vi "全局变量.vi"() -> ()   [LabVIEW 2022 SP3, in "重金属.lvlib"]
panel:
  out "连接配置":T1={"连接类型"=enum."串口", "串口"="", "IP"="192.168.1.205", "PORT"="502"}
  in  "监测值":dbl[](array[numeric])
  in  "因子编码":string[](array[string])=["w20120", "w20115", "w20122", "w20123", "w20121", "w20124", "w20111"]
  in  "参数选择配置":T2 {"通道4" items=["不启用", "铅", "镉", "铜", "锌", "镍", "锰", "汞"]; "通道3" items=["不启用", "铅", "镉", "铜", "锌", "镍", "锰", "汞"]; "通道2" items=["不启用", "铅", "镉", "铜", "锌", "镍", "锰", "汞"]; "通道1" items=["不启用", "铅", "镉", "铜", "锌", "镍", "锰", "汞"]}
  in  "参数名称table":string[](array[string])=["铅", "镉", "铜", "锌"]
  in  "测试时间设置":dbl=3600.0
  in  "运行模式":enum16{"维护模式", "常规模式", "应急模式", "质控模式", "性能测试"}(ring)
  # "w20120\t铅"
  # "w20115\t镉"
  # "w20122\t铜\nw20123\t锌"
  # "铅   镉  铜  锌  镍  锰  汞"
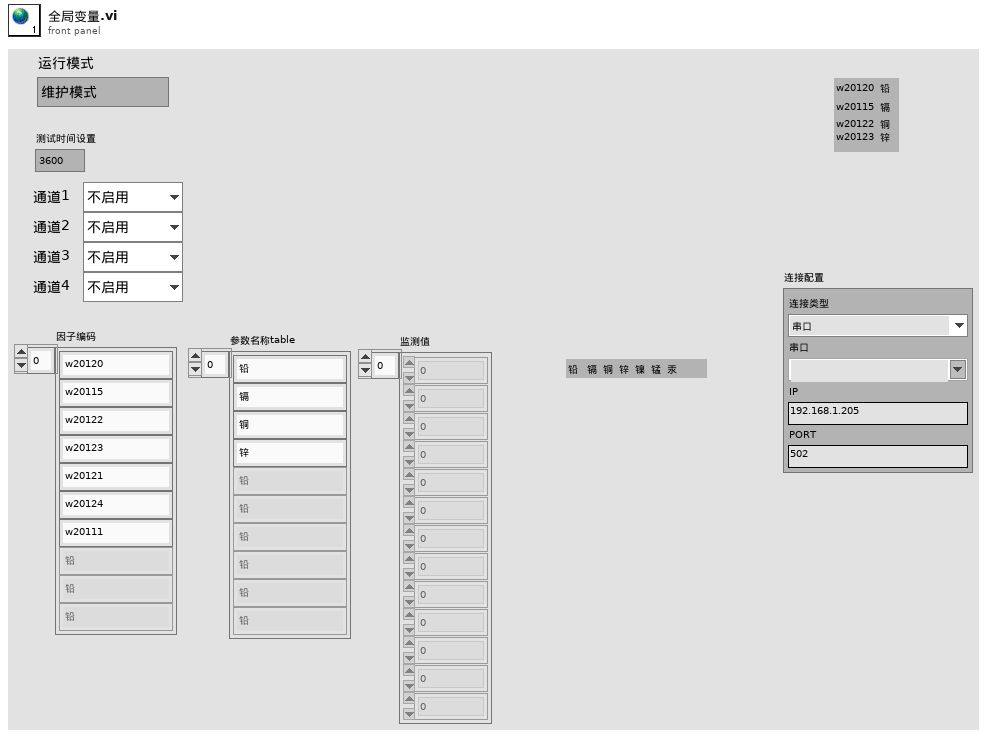
[diagram p1: front panel]
types:
  T1 = cluster{"连接类型":enum16{"串口", "TCP"}, "串口":string, "IP":string, "PORT":string}
  T2 = cluster{"通道1":u16, "通道2":u16, "通道3":u16, "通道4":u16}
diagram:
